vi "KinectToDrive.vi"   [LabVIEW 2011]
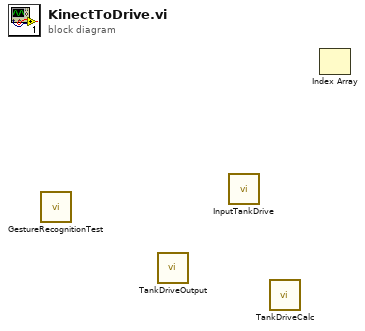
[diagram p0: block diagram]
diagram:
  n1 = call "GestureRecognitionTest.vi"() -> ()  [unwired: 11 in, 1 out]
  n2 = call "TankDriveOutput.vi"() -> ()  [unwired: 16 in]
  n3 = call "InputTankDrive.vi"() -> ()  [unwired: 11 in, 1 out]
  n4 = call "TankDriveCalc.vi"() -> ()  [unwired: 11 in, 1 out]
  n5 = Index Array() -> ()  [unwired: 2 in, 1 out]
